vi "RotToAxisAngle.vi"(2 "Yaw":sgl, 3 "Pitch":sgl) -> (0 "Angle":sgl, 1 "Axis":cluster{"X":sgl, "Y":sgl, "Z":sgl})   [LabVIEW 2015, in "3D Object.lvclass"]
uses:
  3D Object.lvclass
  <vilib>/Analysis/baseanly.llb/Real A x B.vi
  <vilib>/Analysis/NI_AALBase.lvlib
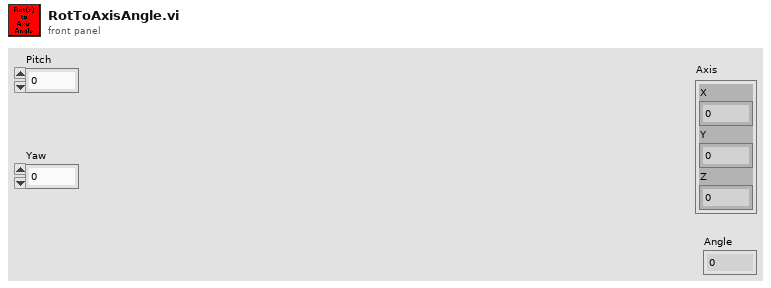
[diagram p1: front panel]
types:
  T1 = typedef "NI_Matrix.lvlib/RealMatrix.ctl" = dbl[][]
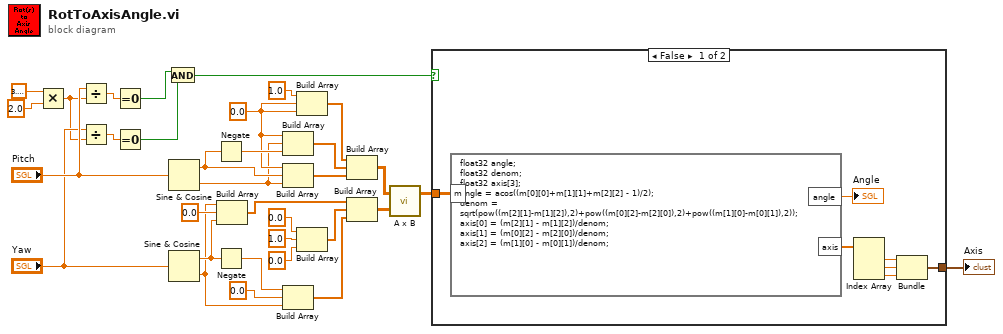
[diagram p0: block diagram]
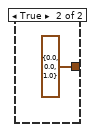
[diagram p2: hidden frame]
diagram:
  w29 = 0.0 ("element")
  n1 = Multiply(x=3.141592653589793, y=2.0) -> (x*y=w5:dbl)
  n2 = Divide(x="Pitch", y=w5) -> (x/y=w4:dbl)
  n3 = Divide(x="Yaw", y=w5) -> (x/y=w3:dbl)
  n4 = Equal To 0?(x=w4) -> (x = 0?=w2:bool)
  n5 = Equal To 0?(x=w3) -> (x = 0?=w1:bool)
  n6 = And(x=w2, y=w1) -> (x .and. y?=w10:bool)
  n7 = Sine & Cosine(0:"Pitch") -> (1:w28:sgl, 2:w27:sgl)
  n8 = Sine & Cosine(0:"Yaw") -> (1:w15:sgl, 2:w13:sgl)
  n9 = Negate(x=w28) -> (-x=w31:sgl)
  n10 = Negate(x=w15) -> (-x=w16:sgl)
  n11 = Build Array(w13, 0.0 ("element"), w15) -> (w20:dbl[])
  n12 = Build Array(w29, w27, w31) -> (w30:dbl[])
  n13 = Build Array(w29, w28, w27) -> (w26:dbl[])
  n14 = Build Array(w16, 0.0 ("element"), w13) -> (w18:dbl[])
  n15 = Build Array(1.0 ("element"), w29, w29) -> (w33:dbl[])
  n16 = Build Array(0.0 ("element"), 1.0 ("element"), 0.0 ("element")) -> (w19:dbl[])
  n17 = Build Array(w33, w30, w26) -> (w25:T1)
  n18 = Build Array(w20, w19, w18) -> (w17:T1)
  n19 = call-poly <vilib>:"A x B.vi"("B"=w17, "A"=w25) -> ("A x B"=w11:T1)  [unwired: 1 out]
  n20 = case shown="False" w10 {
    tunnel: [w35 cluster{sgl, sgl, sgl} {0.0, 0.0, 1.0}] -> w12
    tunnel: w11 -> [w34 _]
    frame False {
      n21 = formula code="float32 angle;\nfloat32 denom;\nfloat32 axis[3];\nangle = acos((m[0][0]+m[1][1]+m[2][2] - 1)/2);\ndenom = sqrt(pow((m[2][1]-m[1][2]),2)+pow((m[0][2]-m[2][0]),2)+pow((m[1][0]-m[0][1]),2));\naxis[0] = (m[2][1] - m[1][2])/denom;\naxis[1] = (m[0][2] - m[2][0])/denom;\naxis[2] = (m[1][0] - m[0][1])/denom;"("m"=w34) -> ("angle"=→"Angle":sgl, "axis"=w39:sgl[])
      n22 = Index Array(array=w39) -> (element #1=w37:sgl, element #2=w38:sgl, element #3=w36:sgl)  [unwired: 3 in]
      n23 = Bundle(w37, w38, w36) -> (w35:cluster{sgl, sgl, sgl})  [unwired: 1 in]
    }
    frame True {
    }
  }
  "Axis" <- w12
